vi "Append Front Panel Image to Report (old string).vi"(0 "report in":refnum<class "NI_report.lvclass">, 1 "alignment (default)":T2, 2 "image format (jpeg)":enum32{"PNG", "JPEG", "GIF"}(ring)=enum."JPEG", 5 "VI":string, 9 "description":string, 11 "error in (no error)":errorcluster, 12 "visible area only?":bool, 13 "MS Office parameters":T1) -> (4 "report out":refnum<class "NI_report.lvclass">, 6 "VI name out":string, 8 "start out (Word)":i32, 10 "end out (Word)":i32, 15 "error out":errorcluster)   [LabVIEW 2015, in "NI_ReportGenerationCore.lvlib"]
doc: "Creates an image of the front panel of the VI you specify in <B>VI</B> and appends it to a report. You can use this polymorphic VI to create a front panel image using a VI path, refnum, or string. The data type you wire to the <B>VI</B> input determines the polymorphic instance to use."
uses:
  <vilib>/Utility/NIReport.llb/NI_ReportGenerationCore.lvlib
  <vilib>/Utility/NIReport.llb/NI_report.lvclass
  <vilib>/Utility/NIReport.llb/HTML Report Image Alignment.ctl
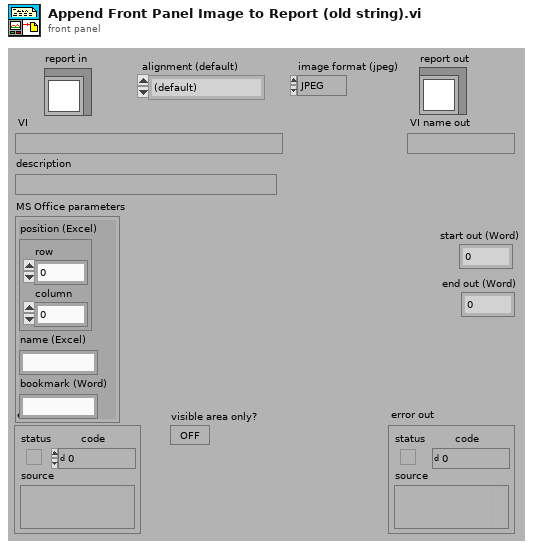
[diagram p1: front panel]
types:
  T1 = cluster{"position (Excel)":cluster{"row":i32, "column":i32}, "name (Excel)":string, "bookmark (Word)":string}
  T2 = typedef "NI_ReportGenerationCore.lvlib/HTML Report Image Alignment.ctl" = enum16{"(default)", "LEFT", "RIGHT", "TOP", "TEXTTOP", "MIDDLE", "ABSMIDDLE", "BASELINE", "BOTTOM", "ABSBOTTOM"}
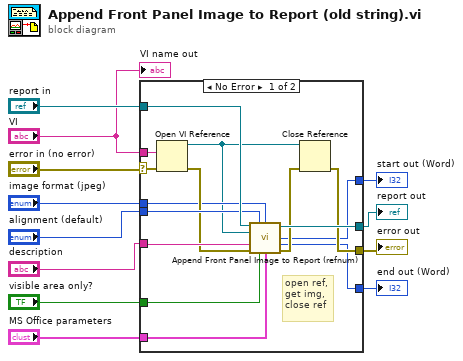
[diagram p0: block diagram]
diagram:
  n1 = case shown="No Error" "error in (no error)" {
    selector: "error in (no error)" -> [w22 w28]
    tunnel: [w15 w28] -> w11
    tunnel: "report in" -> [w27 w29]
    tunnel: "VI" -> [w21 _]
    tunnel: "description" -> [w26 _]
    tunnel: "visible area only?" -> [w25 _]
    tunnel: "alignment (default)" -> [w24 _]
    tunnel: [w23 w29] -> w6
    tunnel: "image format (jpeg)" -> [w19 _]
    tunnel: "MS Office parameters" -> [w18 _]
    tunnel: [w14 _] -> w3
    tunnel: [w13 _] -> w2
    frame No Error {
      # "open ref,\nget img,\nclose ref"
      n2 = Open VI Reference(vi path=w21, error in (no error)=w22) -> (vi reference=w17:refnum<vi>, error out=w20:errorcluster)  [unwired: 4 in]
      n3 = call <vilib>:"Append Front Panel Image to Report (refnum).vi"("report in"=w27, "alignment (default)"=w24, "image format (jpeg)"=w19, "VI"=w17, "description"=w26, "error in (no error)"=w20, "visible area only?"=w25, "MS Office parameters"=w18) -> ("report out"=w23:refnum<class "NI_report.lvclass">, "start out (Word)"=w14:i32, "end out (Word)"=w13:i32, "error out"=w16:errorcluster)  [unwired: 3 in, 1 out]
      n4 = Close Reference(reference=w17, error in (no error)=w16) -> (error out=w15:errorcluster)
    }
    frame Error {
    }
  }
  "error out" <- w11
  "report out" <- w6
  "start out (Word)" <- w3
  "end out (Word)" <- w2
  "VI name out" <- "VI"
